vi "CH1_Comm_Stream.vi"   [LabVIEW 2018]
uses:
  RxTx/RxTx.lvclass
  Stream/Stream.lvclass
  Stream/Stream.lvclass/Stream.ctl
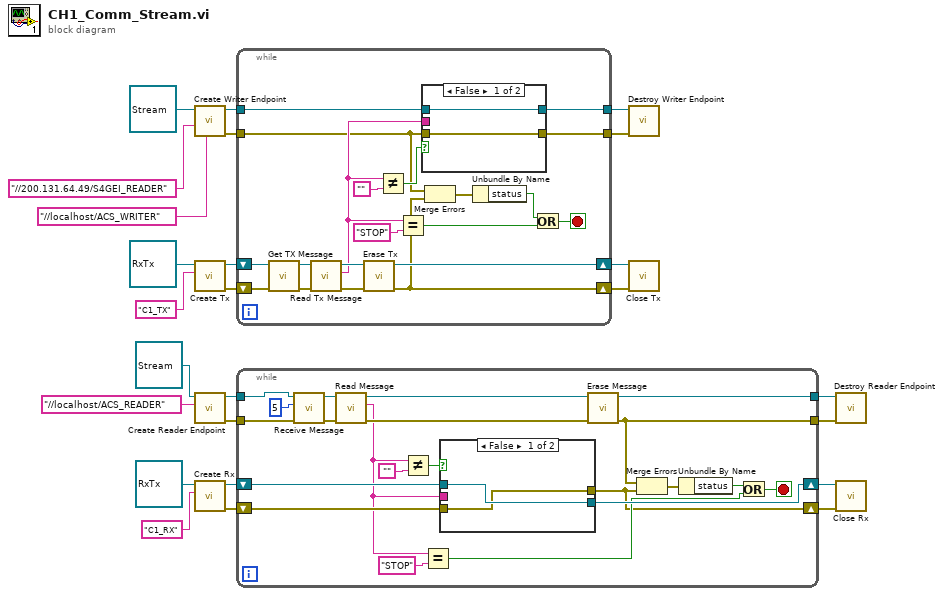
[diagram p0: block diagram]
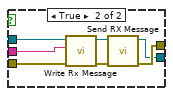
[diagram p2: hidden frame]
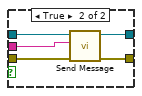
[diagram p3: hidden frame]
diagram:
  n1 = call "Create Writer Endpoint.vi"("writer name"="//localhost/ACS_WRITER" ("reader name"), "reader name"="//200.131.64.49/S4GEI_READER", "Stream in"=refnum<class "Stream.lvclass"> refnum) -> ("error out"=w10:errorcluster, "Stream out"=w11:refnum<class "Stream.lvclass">)  [unwired: 7 in]
  n2 = call "Create Tx.vi"("Writer Name"="C1_TX", "RxTx in"=refnum<class "RxTx.lvclass"> refnum ("RxTx.lvclass")) -> ("error out"=w24:errorcluster, "RxTx out"=w25:refnum<class "RxTx.lvclass">)  [unwired: 8 in]
  n3 = call "Create Reader Endpoint.vi"("reader name"="//localhost/ACS_READER", "Stream in"=refnum<class "Stream.lvclass"> refnum) -> ("error out"=w14:errorcluster, "Stream out"=w15:refnum<class "Stream.lvclass">)  [unwired: 8 in]
  n4 = call "Create Rx.vi"("Reader Name"="C1_RX", "RxTx in"=refnum<class "RxTx.lvclass"> refnum ("RxTx.lvclass")) -> ("error out"=w20:errorcluster, "RxTx out"=w21:refnum<class "RxTx.lvclass">)  [unwired: 8 in]
  n5 = while {
    shift-right: [w39] -> w22
    shift-left: w25 -> [w45]
    shift-right: [w28] -> w23
    shift-left: w24 -> [w44]
    tunnel: w11 -> [w36]
    tunnel: w10 -> [w27]
    tunnel: [w35] -> w9
    tunnel: [w34] -> w8
    stop <- w29 stop-if-true
    n6 = call "Get TX Message.vi"("error in (no error)"=w44, "RxTx in"=w45) -> ("error out"=w42:errorcluster, "RxTx out"=w43:refnum<class "RxTx.lvclass">)  [unwired: 8 in]
    n7 = call "Read Tx Message.vi"("error in (no error)"=w42, "RxTx in"=w43) -> ("error out"=w41:errorcluster, "Tx Message"=w33:string, "RxTx out"=w40:refnum<class "RxTx.lvclass">)  [unwired: 7 in]
    n8 = call "Erase Tx.vi"("error in (no error)"=w41, "RxTx in"=w40) -> ("error out"=w28:errorcluster, "RxTx out"=w39:refnum<class "RxTx.lvclass">)  [unwired: 8 in]
    n9 = Not Equal?(x=w33, y="") -> (x != y?=w37:bool)
    n10 = Equal?(x=w33, y="STOP") -> (x = y?=w31:bool)
    n11 = case shown="False" w37 {
      tunnel: w33 -> [_ w52]
      tunnel: w36 -> [w47 w51]
      tunnel: w27 -> [w46 w50]
      tunnel: [w46 w49] -> w35
      tunnel: [w47 w48] -> w34
      frame False {
      }
      frame True {
        n12 = call "Send Message.vi"("error in (no error)"=w50, "Message"=w52, "Stream in"=w51) -> ("error out"=w49:errorcluster, "Stream out"=w48:refnum<class "Stream.lvclass">)  [unwired: 7 in]
      }
    }
    n13 = Merge Errors(w27, w28) -> (w26:errorcluster)
    n14 = Unbundle By Name(w26) -> ("status"=w30:bool)
    n15 = Or(x=w30, y=w31) -> (x .or. y?=w29:bool)
  }
  n16 = while {
    shift-right: [w71] -> w18
    shift-left: w21 -> [w73]
    shift-right: [w57] -> w19
    shift-left: w20 -> [w72]
    tunnel: w15 -> [w70]
    tunnel: w14 -> [w69]
    tunnel: [w63] -> w13
    tunnel: [w56] -> w12
    stop <- w53 stop-if-true
    n17 = call "Receive Message.vi"("error in (no error)"=w69, "timeout ms"=5, "Stream in"=w70) -> ("error out"=w66:errorcluster, "Stream out"=w67:refnum<class "Stream.lvclass">)  [unwired: 7 in]
    n18 = call "Read Message.vi"("error in (no error)"=w66, "Stream in"=w67) -> ("error out"=w64:errorcluster, "Message"=w59:string, "Stream out"=w65:refnum<class "Stream.lvclass">)  [unwired: 7 in]
    n19 = Not Equal?(x=w59, y="") -> (x != y?=w61:bool)
    n20 = Equal?(x=w59, y="STOP" ("reader name")) -> (x = y?=w58:bool)
    n21 = case shown="False" w61 {
      tunnel: w73 -> [w75 w82]
      tunnel: w72 -> [w74 w79]
      tunnel: [w74 w78] -> w57
      tunnel: [w75 w77] -> w71
      tunnel: w59 -> [_ w76]
      frame False {
      }
      frame True {
        n22 = call "Write Rx Message.vi"("error in (no error)"=w79, "Rx Message"=w76, "RxTx in"=w82) -> ("error out"=w80:errorcluster, "RxTx out"=w81:refnum<class "RxTx.lvclass">)  [unwired: 7 in]
        n23 = call "Send RX Message.vi"("error in (no error)"=w80, "RxTx in"=w81) -> ("error out"=w78:errorcluster, "RxTx out"=w77:refnum<class "RxTx.lvclass">)  [unwired: 8 in]
      }
    }
    n24 = call "Erase Message.vi"("error in (no error)"=w64, "Stream in"=w65) -> ("error out"=w56:errorcluster, "Stream out"=w63:refnum<class "Stream.lvclass">)  [unwired: 8 in]
    n25 = Merge Errors(w56, w57) -> (w55:errorcluster)
    n26 = Unbundle By Name(w55) -> ("status"=w54:bool)
    n27 = Or(x=w54, y=w58) -> (x .or. y?=w53:bool)
  }
  n28 = call "Destroy Writer Endpoint.vi"("error in (no error)"=w9, "Stream in"=w8) -> ()  [unwired: 8 in, 2 out]
  n29 = call "Close Tx.vi"("error in (no error)"=w23, "RxTx in"=w22) -> ()  [unwired: 8 in, 2 out]
  n30 = call "Destroy Reader Endpoint.vi"("error in (no error)"=w12, "Stream in"=w13) -> ()  [unwired: 8 in, 2 out]
  n31 = call "Close Rx.vi"("error in (no error)"=w19, "RxTx in"=w18) -> ()  [unwired: 8 in, 2 out]
